vi "PNA_VISA_WRITE-READ.vi"(0 "Session In":refnum<visa-resource-name>="TCPIP0::K-N5224B-41806.localdomain::inst0::INSTR", 1 "Wcmd":string="sens:corr:coll:guid:conn:port1", 4 "Rcmd":string="sens:corr:coll:guid:conn:port1?", 5 "error in":errorcluster {"code" format="%.0x"}, 6 "Timeout":u32=3000, 7 "READ":bool, 9 "Check Errors(t)":bool=TRUE, 13 "WRITE":bool) -> (12 "Out":string="\"2.92 mm female\"", 14 "Session Out":refnum<visa-resource-name>="TCPIP0::K-N5224B-41806.localdomain::inst0::INSTR", 19 "error out":errorcluster {"code" format="%.0x"})   [LabVIEW 2018]
doc: "VISA READ/WRITE Vi"
panel:
  out "Error Code":i32[](array[numeric])
  out "SCPI":string="sens:corr:coll:guid:conn:port1 \"2.92 mm female\""
  in  "Wcmd Val":string="\"2.92 mm female\""
  out "Error Message":string="+0,\"No error\"\r\n"
  # "sens:corr:coll:guid:init"
  # "sens:corr:coll:guid:conn:port1 \"2.92mm female\""
  # "sens:corr:coll:guid:ckit:port1 \"N4692-60003 ECal 13203\""
  # "sens:corr:coll:guid:init"
  # "sens:corr:coll:guid:steps?"
  # "+1"
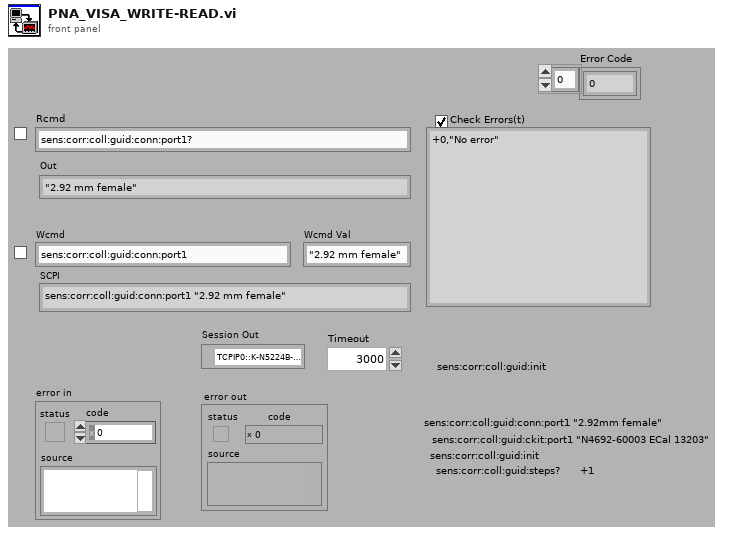
[diagram p1: front panel]
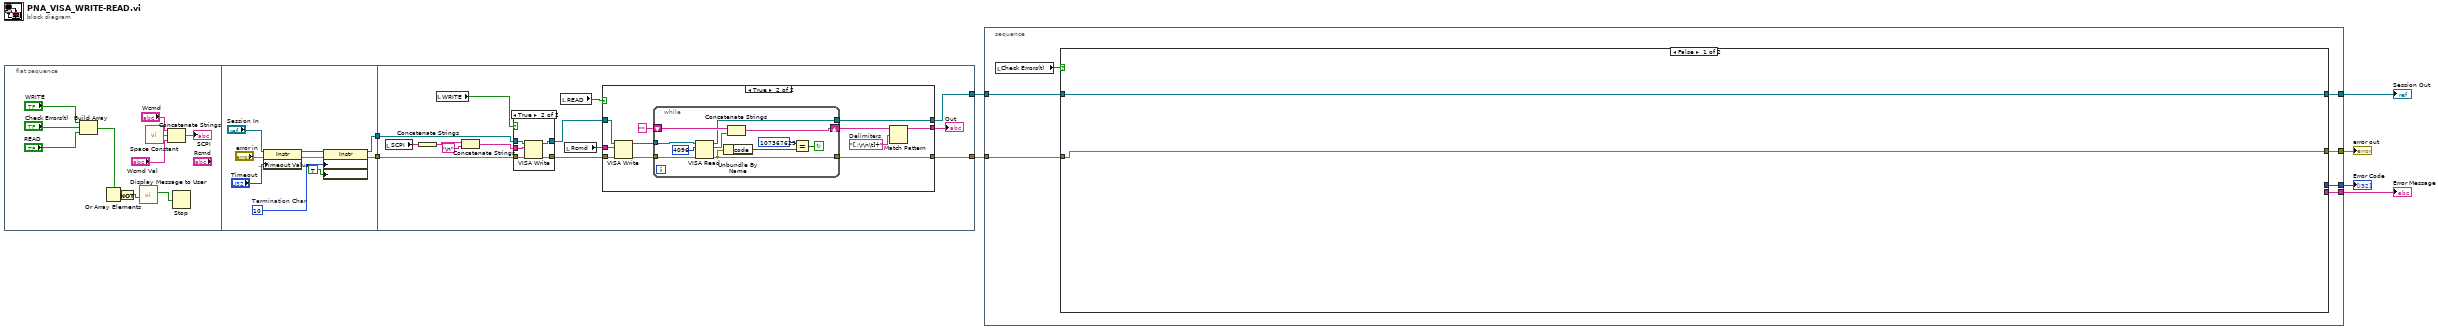
[diagram p0: block diagram]
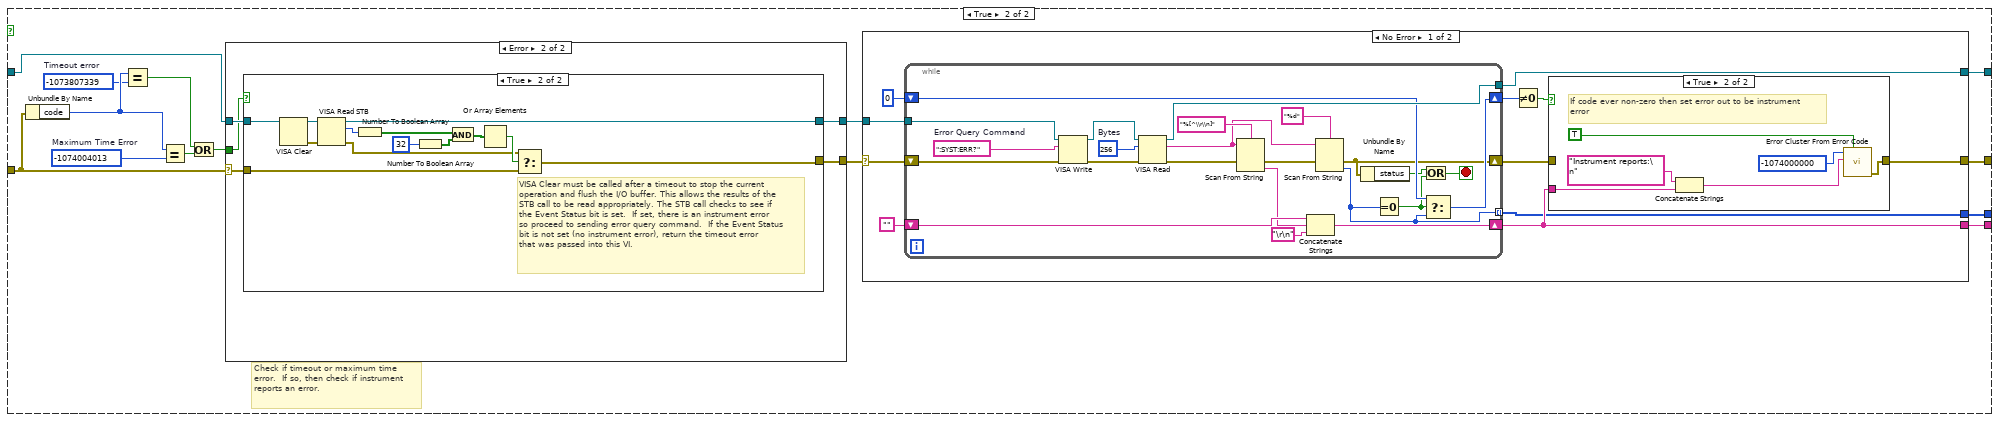
[diagram p2: hidden frame]
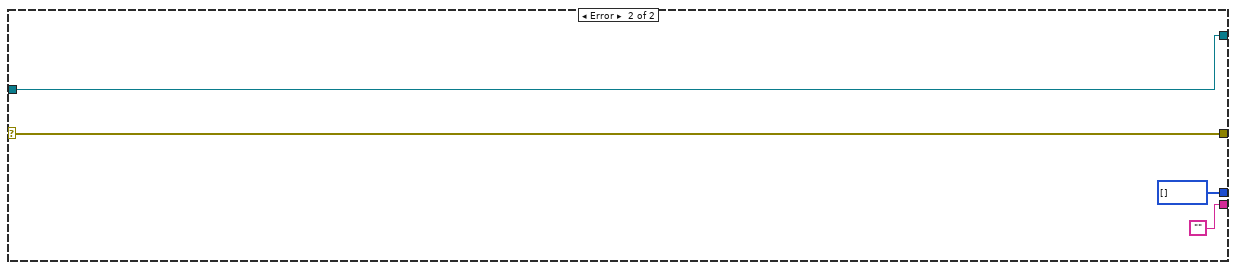
[diagram p6: hidden frame]
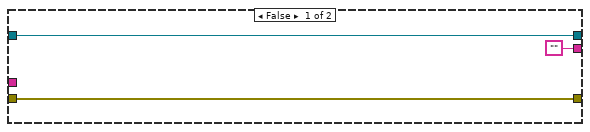
[diagram p8: hidden frame]
diagram:
  n1 = flat-sequence {
    tunnel: [w24] -> w8
    tunnel: [w20] -> w7
    tunnel: w8 -> [w38]
    tunnel: w7 -> [w37]
    tunnel: [w32] -> w3
    tunnel: [w31] -> w2
    frame #0 {
      n2 = Build Array("WRITE", "Check Errors(t)", "READ") -> (w12:bool[])
      n3 = Or Array Elements(Boolean array=w12) -> (logical OR=w11:bool)
      n4 = Not(x=w11) -> (.not. x?=w10:bool)
      n5 = call "Display Message to User"("Enable"=w10) -> ("OK"=w9:bool)  [unwired: 9 in, 1 out]
      n6 = call <vilib>:"Space Constant.vi"() -> ("String"=w17:string)
      n7 = Concatenate Strings("Wcmd", w17, "Wcmd Val") -> (→"SCPI":string)
      n8 = Stop(stop? (T)=w9) -> ()
    }
    frame #1 {
      w23 = u8 10  # Termination Char
      n9 = property class="Instr"(reference="Session In", error in="error in", "General Settings:Timeout Value"="Timeout") -> (reference out=w22:refnum<visa-resource-name>, error out=w25:errorcluster)
      n10 = property class="Instr"(reference=w22, error in=w25, "Message Based Settings:Termination Character"=w23, "Message Based Settings:Termination Character Enable"=TRUE ("enable")) -> (reference out=w20:refnum<visa-resource-name>, error out=w24:errorcluster)
    }
    frame #2 {
      n11 = local read "SCPI"() -> (w33:string)
      n12 = Concatenate Strings(w33) -> (w36:string)
      n13 = local read "WRITE"() -> (w30:bool)
      n14 = Concatenate Strings(w36, "\n" ("StaticText")) -> (w34:string)
      n15 = case shown="True" w30 {
        tunnel: w38 -> [w43 w49]
        tunnel: [w43 w48] -> w41
        tunnel: w34 -> [_ w47]
        tunnel: w37 -> [w44 w46]
        tunnel: [w44 w45] -> w40
        frame False {
        }
        frame True {
          n16 = VISA Write(VISA resource name=w46, write buffer=w47, error in (no error)=w49) -> (VISA resource name out=w45:refnum<visa-resource-name>, error out=w48:errorcluster)  [unwired: 1 out]
        }
      }
      n17 = local read "READ"() -> (w29:bool)
      n18 = local read "Rcmd"() -> (w39:string)
      n19 = case shown="True" w29 {
        tunnel: w41 -> [w51 w63]
        tunnel: w39 -> [_ w59]
        tunnel: ["" w58] -> w42
        tunnel: w40 -> [w52 w55]
        tunnel: [w52 w54] -> w31
        tunnel: [w51 w53] -> w32
        frame False {
        }
        frame True {
          w57 = "[,;\r\n\t]+"  # Delimiters
          n20 = VISA Write(VISA resource name=w55, write buffer=w59, error in (no error)=w63) -> (VISA resource name out=w62:refnum<visa-resource-name>, error out=w61:errorcluster)  [unwired: 1 out]
          n21 = while {
            tunnel: w62 -> [w71]
            shift-right: [w65] -> w56
            shift-left: "" -> [w70]
            tunnel: w61 -> [w68]
            tunnel: [w67] -> w53
            tunnel: [w64] -> w54
            stop <- w66 continue-if-true
            n22 = VISA Read(VISA resource name=w71, byte count=u32 4096 ("byte count (0)"), error in (no error)=w68) -> (VISA resource name out=w64:refnum<visa-resource-name>, read buffer=w69:string, error out=w67:errorcluster)  [unwired: 1 out]
            n23 = Unbundle By Name(w67) -> ("code"=w73:i32)
            n24 = Concatenate Strings(w70, w69) -> (w65:string)
            n25 = Equal?(x=1073676294, y=w73) -> (x = y?=w66:bool)
          }
          n26 = Match Pattern(string=w56, regular expression=w57) -> (before substring=w58:string)  [unwired: 4 out]
        }
      }
      "Out" <- w42
    }
  }
  n27 = stacked-sequence {
    tunnel: [w77] -> w5
    tunnel: [w78] -> w6
    tunnel: [w79] -> w1
    tunnel: [w76] -> w4
    tunnel: w3 -> [w81]
    tunnel: w2 -> [w80]
    frame #0 {
      n28 = local read "Check Errors(t)"() -> (w75:bool)
      n29 = case shown="False" w75 {
        tunnel: w81 -> [w83 w97]
        tunnel: w80 -> [w82 w90]
        tunnel: [_ w87] -> w79
        tunnel: [_ w86] -> w78
        tunnel: [w83 w85] -> w77
        tunnel: [w82 w84] -> w76
        frame False {
        }
        frame True {
          w93 = -1074004013  # Maximum Time Error
          w91 = -1073807339  # Timeout error
          # "Check if timeout or maximum time error.  If so, then check if instrument reports an error."
          n30 = Unbundle By Name(w97) -> ("code"=w92:i32)
          n31 = Equal?(x=w92, y=w91) -> (x = y?=w95:bool)
          n32 = Equal?(x=w92, y=w93) -> (x = y?=w94:bool)
          n33 = Or(x=w95, y=w94) -> (x .or. y?=w96:bool)
          n34 = case shown="Error" w97 {
            selector: w97 -> [w98 w102]
            tunnel: w90 -> [w99 w104]
            tunnel: [w99 w103] -> w89
            tunnel: [w98 w101] -> w88
            tunnel: w96 -> [_ w100]
            frame No Error {
            }
            frame Error {
              n35 = case shown="True" w100 {
                tunnel: w104 -> [w106 w112]
                tunnel: [w106 w109] -> w103
                tunnel: w102 -> [w105 w115]
                tunnel: [w105 w114] -> w101
                frame False {
                  # "Error code not a timeout, so best to pass on to user."
                }
                frame True {
                  # "VISA Clear must be called after a timeout to stop the current operation and flush the I/O buffer. This allows the results of the  STB call to be read appropriately. The STB call checks to see if the Event Status bit is set.  If set, there is an instrument error so proceed to sending error query command.  If the Event Status bit is not set (no instrument error), return the timeout error that was passed into this VI."
                  n36 = VISA Clear(VISA resource name=w112) -> (VISA resource name out=w111:refnum<visa-resource-name>, error out=w110:errorcluster)  [unwired: 1 in]
                  n37 = VISA Read STB(8:w110, 11:w111) -> (0:w108:errorcluster, 2:w107:u16, 3:w109:refnum<visa-resource-name>)
                  n38 = Number To Boolean Array(number=w107) -> (Boolean array=w116:bool[])
                  n39 = Number To Boolean Array(number=32) -> (Boolean array=w118:bool[])
                  n40 = And(x=w116, y=w118) -> (x .and. y?=w117:bool[])
                  n41 = Or Array Elements(Boolean array=w117) -> (logical OR=w113:bool)
                  n42 = Select(t=w108, s=w113, f=w115) -> (s? t:f=w114:errorcluster)
                }
              }
            }
          }
          n43 = case shown="No Error" w88 {
            selector: w88 -> [w121 w161]
            tunnel: [w130 w164] -> w84
            tunnel: w89 -> [w129 w164]
            tunnel: [w120 w161] -> w85
            tunnel: [w124 ""] -> w86
            tunnel: [w123 i32[] []] -> w87
            frame No Error {
              n44 = while {
                tunnel: [w160] -> w130
                tunnel: w129 -> [w159]
                shift-right: [w147] -> w124
                shift-left: "" -> [w150]
                shift-right: [w145] -> w125
                shift-left: 0 -> [w146]
                shift-right: [w143] -> w122
                shift-left: w121 -> [w144]
                tunnel: [w138] -> w123 mode=indexing
                stop <- w153 stop-if-true
                w157 = u32 256  # Bytes
                w155 = ":SYST:ERR?"  # Error Query Command
                n45 = VISA Write(VISA resource name=w159, write buffer=w155, error in (no error)=w144) -> (VISA resource name out=w158:refnum<visa-resource-name>, error out=w156:errorcluster)  [unwired: 1 out]
                n46 = VISA Read(VISA resource name=w158, byte count=w157, error in (no error)=w156) -> (VISA resource name out=w160:refnum<visa-resource-name>, read buffer=w151:string, error out=w142:errorcluster)  [unwired: 1 out]
                n47 = Scan From String(format string="%[^\\r\\n]", input string=w151, error in=w142) -> (error out=w141:errorcluster, output 1=w148:string)  [unwired: 2 in, 2 out]
                n48 = Concatenate Strings(w150, w148, "\r\n") -> (w147:string)
                n49 = Scan From String(format string="%d", input string=w151, error in=w141) -> (error out=w143:errorcluster, output 1=w138:i32)  [unwired: 2 in, 2 out]
                n50 = Unbundle By Name(w143) -> ("status"=w140:bool)
                n51 = Equal To 0?(x=w138) -> (x = 0?=w139:bool)
                n52 = Or(x=w140, y=w139) -> (x .or. y?=w153:bool)
                n53 = Select(t=w146, s=w139, f=w138) -> (s? t:f=w145:i32)
              }
              n54 = Not Equal To 0?(x=w125) -> (x != 0?=w126:bool)
              n55 = case shown="True" w126 {
                tunnel: w124 -> [_ w136]
                tunnel: [w131 w132] -> w120
                tunnel: w122 -> [w131 _]
                frame False {
                }
                frame True {
                  # "If code ever non-zero then set error out to be instrument error"
                  n56 = Concatenate Strings("Instrument reports:\n" ("Source"), w136) -> (w133:string)
                  n57 = call <vilib>:"Error Cluster From Error Code.vi"("show call chain? (False)"=TRUE, "error message (\"\")"=w133, "error code (0)"=-1074000000 ("Code")) -> ("error out"=w132:errorcluster)  [unwired: 6 in]
                }
              }
            }
            frame Error {
            }
          }
        }
      }
    }
  }
  "Session Out" <- w4
  "error out" <- w5
  "Error Message" <- w6
  "Error Code" <- w1
